vi "Vacuum Pumps.vi"(0 "CloseVi?":bool) -> ()   [LabVIEW 2011]
uses:
  Controls/Gate Valve - Horizontal.ctl
  Controls/Gate Valve - Vertical.ctl
  GlobalVariables.vi
panel:
  in  "Open Ion Guage VI":bool
  out "Boolean 8":bool
  in  "108":T1
  in  "107":T2
  in  "101":T1
  in  "109":T1
  in  "111":T1
  in  "105":T2
  in  "117":T2
  in  "115":T2
  out "Boolean 9":bool
  out "Boolean 18":bool
  out "Boolean 17":bool
  out "Boolean 5":bool
  out "GP275 Conv.":sgl format="%#_5e"
  in  "Open (100)":bool
  in  "Close (99)":bool
  in  "TP":bool
  out "Boolean 16":bool
  out "Boolean 15":bool
  out "Boolean 14":bool
  out "Ion Guage":dbl format="%#_5e"
  out "Boolean 13":bool
  out "Boolean 11":bool
  out "Boolean 10":bool
  in  "Turbo Pump":bool=TRUE
  out "Boolean 7":bool
  out "Boolean 6":bool
  out "Boolean 4":bool
  out "Boolean 3":bool
  out "Boolean 2":bool
  out "Boolean":bool
  out "94":dbl format="%#_3e"
  out "93":dbl format="%#_3e"
  out "92":dbl format="%#_3e"
  out "91":dbl format="%#_3e"
  out "90":dbl format="%#_3e"
  in  "BAR94 Byte 2":u8
  in  "BAR94 Byte 1":u8
  in  "BAR93 Byte 2":u8
  in  "BAR93 Byte 1":u8
  in  "BAR92 Byte 2":u8
  in  "BAR92 Byte 1":u8
  in  "BAR91 Byte 2":u8
  in  "BAR91 Byte 1":u8
  in  "BAR90 Byte 2":u8
  in  "BAR90 Byte 1":u8
  in  "TT":bool
  in  "GP354 Input Byte 2":u8
  in  "GP354 Input Byte 1":u8
  in  "GP275 Input Byte 1":u8
  in  "GP275 Input Byte 2":u8
  in  "GP275 Input Byte 3":u8
  in  "GP275 Input Byte 4":u8
  in  "Scroll Pump":bool=TRUE
  in  "Close":bool
  out "Boolean 12":bool
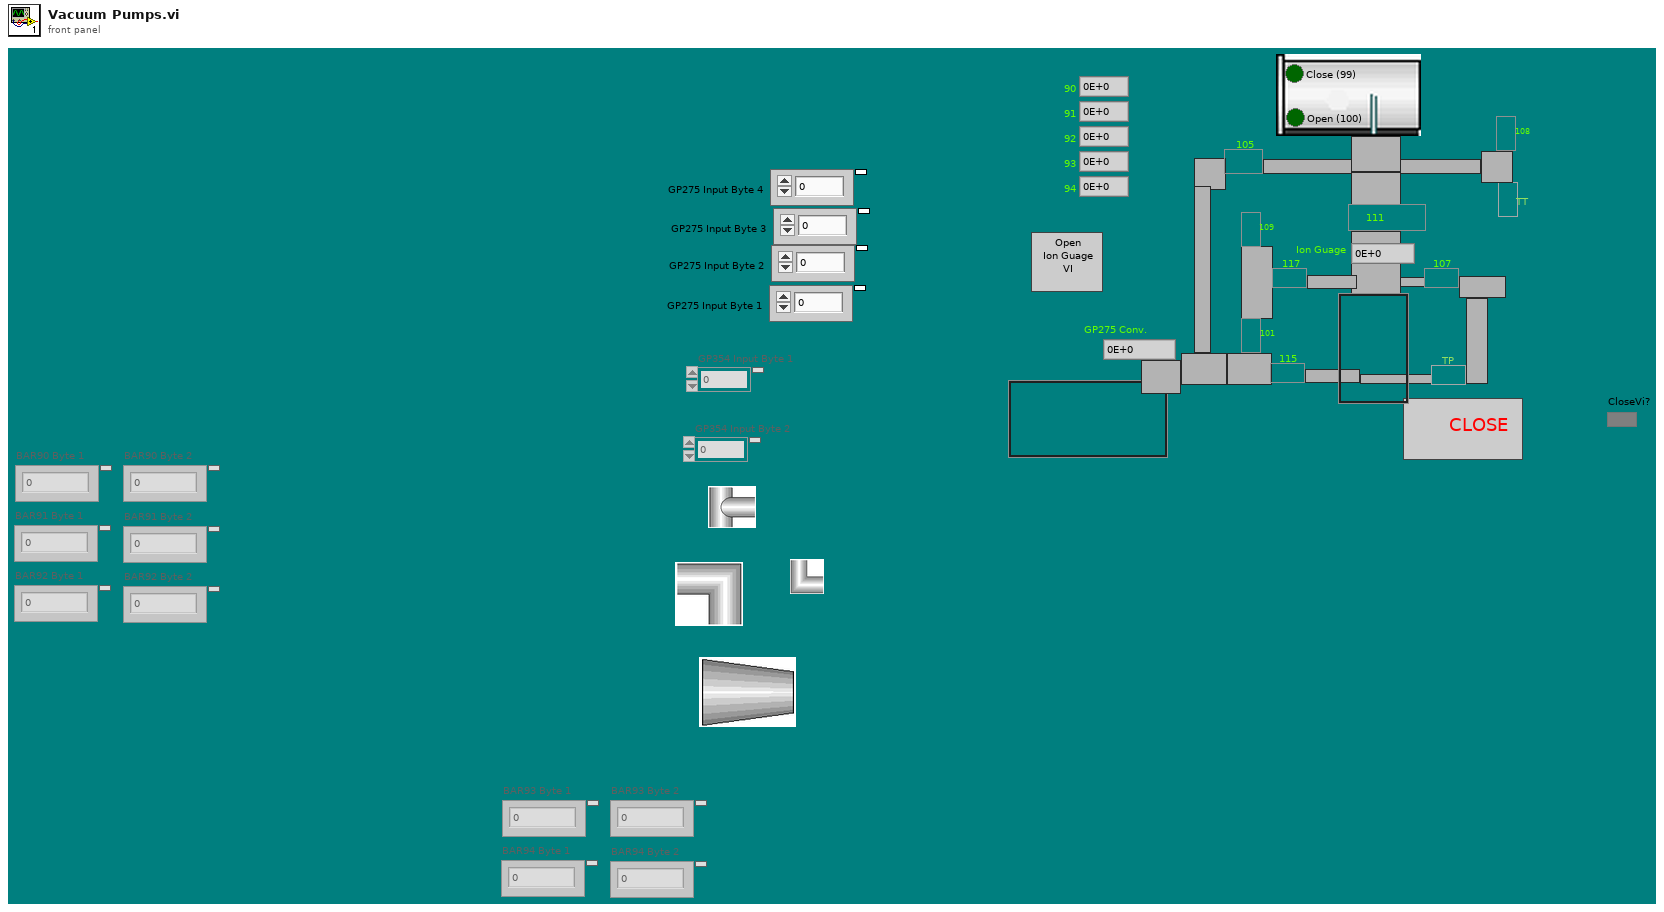
[diagram p1: front panel]
types:
  T1 = typedef "Gate Valve - Vertical.ctl" = bool
  T2 = typedef "Gate Valve - Horizontal.ctl" = bool
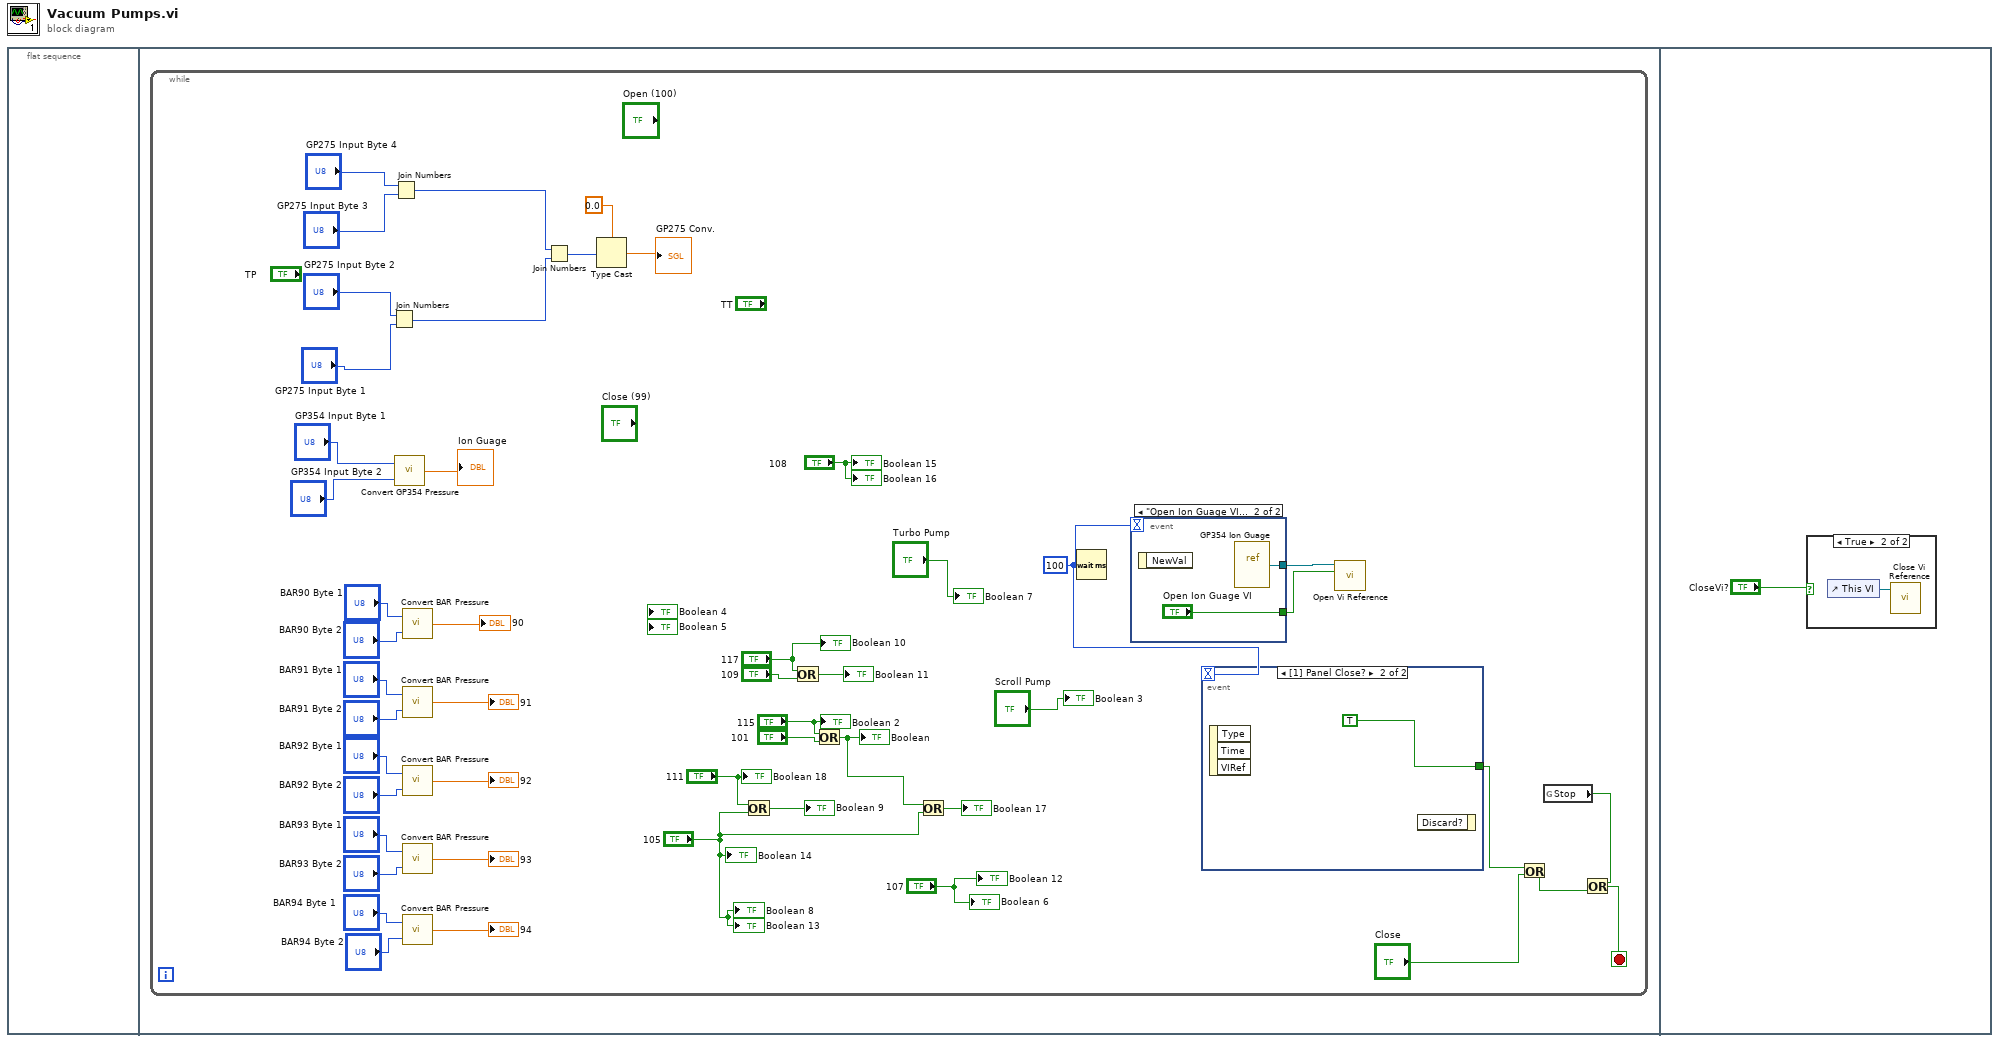
[diagram p0: block diagram]
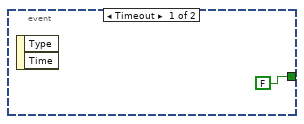
[diagram p2: hidden frame]
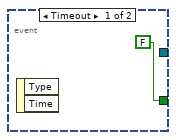
[diagram p3: hidden frame]
diagram:
  n1 = flat-sequence {
    frame #0 {
    }
    frame #1 {
      n2 = while {
        stop <- w7 stop-if-true
        w6 = u32 100 ("milliseconds to wait")
        n3 = Join Numbers(hi="GP275 Input Byte 2", lo="GP275 Input Byte 1") -> ((hi.lo)=w48:u16)
        n4 = Join Numbers(hi="GP275 Input Byte 4", lo="GP275 Input Byte 3") -> ((hi.lo)=w47:u16)
        n5 = call "Convert GP354 Pressure.vi"("Input Byte 2"="GP354 Input Byte 2", "Input Byte 1"="GP354 Input Byte 1") -> ("Pressure"=→"Ion Guage":dbl)
        n6 = call "Convert BAR Pressure.vi"("Input Byte 2"="BAR90 Byte 2", "Input Byte 1"="BAR90 Byte 1") -> ("Pressure"=→"90":dbl)
        n7 = call "Convert BAR Pressure.vi"("Input Byte 2"="BAR91 Byte 2", "Input Byte 1"="BAR91 Byte 1") -> ("Pressure"=→"91":dbl)
        n8 = call "Convert BAR Pressure.vi"("Input Byte 2"="BAR92 Byte 2", "Input Byte 1"="BAR92 Byte 1") -> ("Pressure"=→"92":dbl)
        n9 = call "Convert BAR Pressure.vi"("Input Byte 2"="BAR93 Byte 2", "Input Byte 1"="BAR93 Byte 1") -> ("Pressure"=→"93":dbl)
        n10 = call "Convert BAR Pressure.vi"("Input Byte 2"="BAR94 Byte 2", "Input Byte 1"="BAR94 Byte 1") -> ("Pressure"=→"94":dbl)
        n11 = Join Numbers(hi=w47, lo=w48) -> ((hi.lo)=w46:u32)
        n12 = Type Cast(type=sgl 0.0, x=w46) -> (*(type *) &x=→"GP275 Conv.":sgl)
        n13 = Or(x="111", y="105") -> (x .or. y?=→"Boolean 9":T1)
        n14 = Or(x="117", y="109") -> (x .or. y?=→"Boolean 11":T2)
        n15 = Or(x="115", y="101") -> (x .or. y?=w10:T2)
        "Boolean" <- w10
        n16 = Or(x=w10, y="105") -> (x .or. y?=→"Boolean 17":T2)
        n17 = Wait (ms)(milliseconds to wait=w6) -> ()  [unwired: 1 out]
        n18 = event shown="[1] \"Open Ion Guage VI\": Value Change" {
          selector: _ -> [_ _]
          dyn-events: _ -> [_ _]
          timeout: w6 -> [_ _]
          tunnel: [FALSE ("Open Festo VI") "Open Ion Guage VI"] -> w1
          tunnel: [_ w53] -> w2
          event Timeout {
            n19 = event-data() -> ()  [unwired: 1 in, 2 out]
          }
          event "Open Ion Guage VI": Value Change {
            n20 = event-data() -> ()  [unwired: 1 in, 1 out]
            n21 = vi-ref "GP354 Ion Guage.vi"() -> (w53:refnum<vi>)
          }
        }
        n22 = event shown="[1] Panel Close?" {
          selector: _ -> [_ _]
          dyn-events: _ -> [_ _]
          timeout: w6 -> [_ _]
          tunnel: [FALSE ("y") TRUE ("y")] -> w3
          event Timeout {
            n23 = event-data() -> ()  [unwired: 1 in, 2 out]
          }
          event Panel Close? {
            n24 = event-data() -> ()  [unwired: 1 in, 3 out]
            n25 = event-data() -> ()  [unwired: 2 in, 1 out]
          }
        }
        n26 = call "Open Vi Reference.vi"("RunVi"=w1, "reference"=w2) -> ()  [unwired: 2 in, 2 out]
        n27 = Or(x=w3, y="Close") -> (x .or. y?=w5:bool)
        n28 = global read "GlobalVariables.vi" "Stop"() -> (w8:bool)
        n29 = Or(x=w8, y=w5) -> (x .or. y?=w7:bool)
        "Boolean 2" <- "115"
        "Boolean 3" <- "Scroll Pump"
        "Boolean 6" <- "107"
        "Boolean 7" <- "Turbo Pump"
        "Boolean 10" <- "117"
        "Boolean 12" <- "107"
        "Boolean 15" <- "108"
        "Boolean 16" <- "108"
        "Boolean 8" <- "105"
        "Boolean 13" <- "105"
        "Boolean 14" <- "105"
        "Boolean 18" <- "111"
      }
    }
    frame #2 {
      n30 = case shown="True" "CloseVi?" {
        frame False {
        }
        frame True {
          n31 = control-ref of="This VI"() -> (w56:refnum<vi>)
          n32 = call "Close Vi Reference.vi"("reference"=w56) -> ()  [unwired: 9 in, 2 out]
        }
      }
    }
  }
